vi "FindTreeKey.vi"(8 "error in (no error)":errorcluster, 10 "Key":T3, 11 "Map":T4) -> (0 "error out":errorcluster, 1 "How rotated?":i8[](array[numeric]), 2 "DecisionRecord":T1, 3 "IsFound?":bool)   [LabVIEW 2020]
uses:
  controls/DecisionTree.ctl
  controls/Gameboard Data.ctl
  controls/DecisionTreeRecord.ctl
  controls/Player.ctl
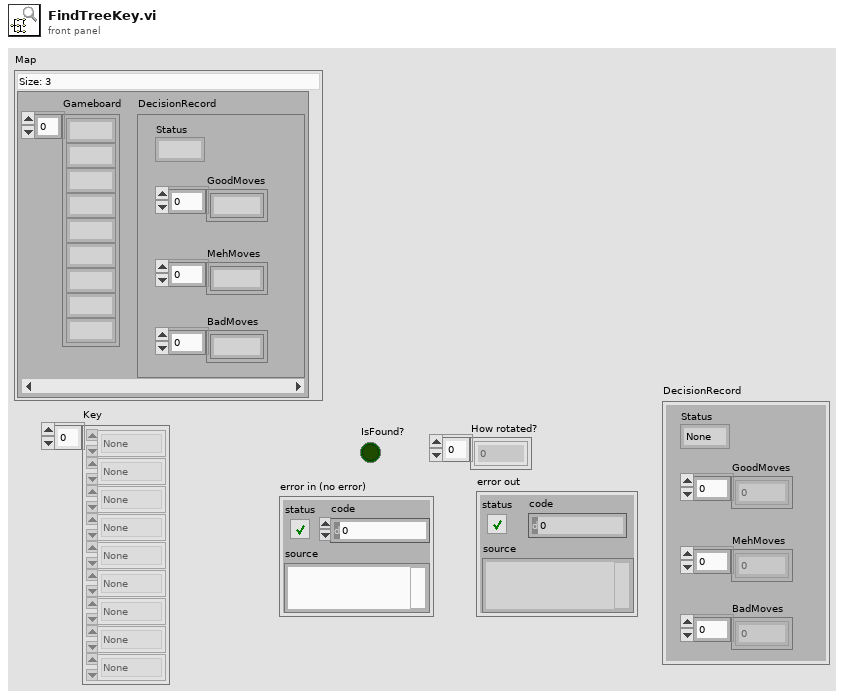
[diagram p1: front panel]
types:
  T1 = typedef "DecisionTreeRecord.ctl" = cluster{"Status":T2, "GoodMoves":i8[], "MehMoves":i8[], "BadMoves":i8[]}
  T2 = typedef "Player.ctl" = enum16{"None", "Player 1", "Player 2"}
  T3 = typedef "Gameboard Data.ctl" = enum16{"None", "Player 1", "Player 2"}[]
  T4 = typedef "DecisionTree.ctl" = map{T3, T1}
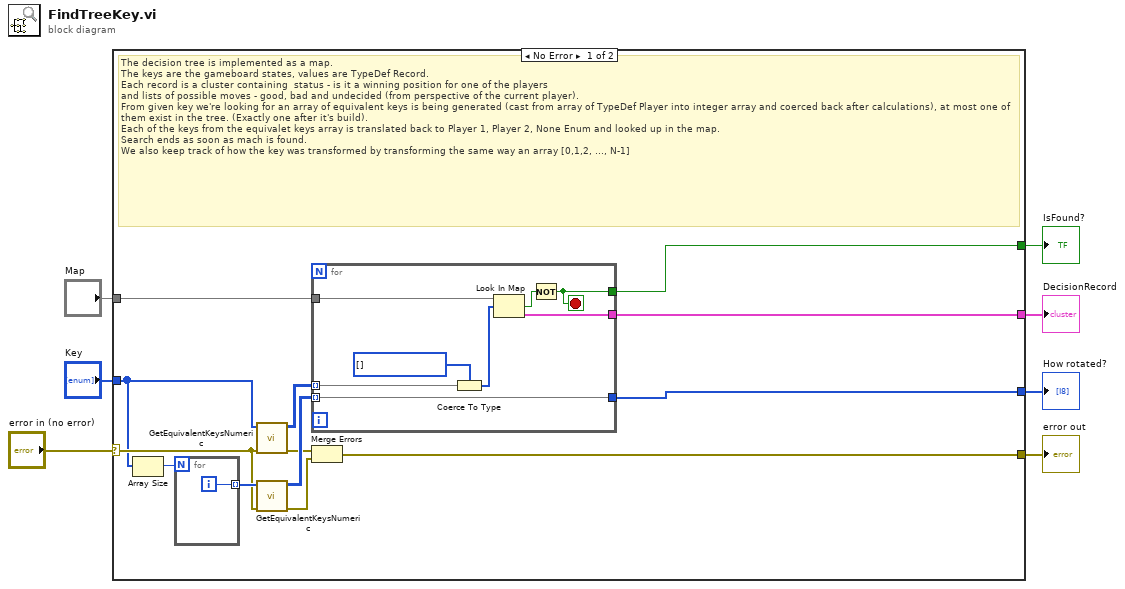
[diagram p0: block diagram]
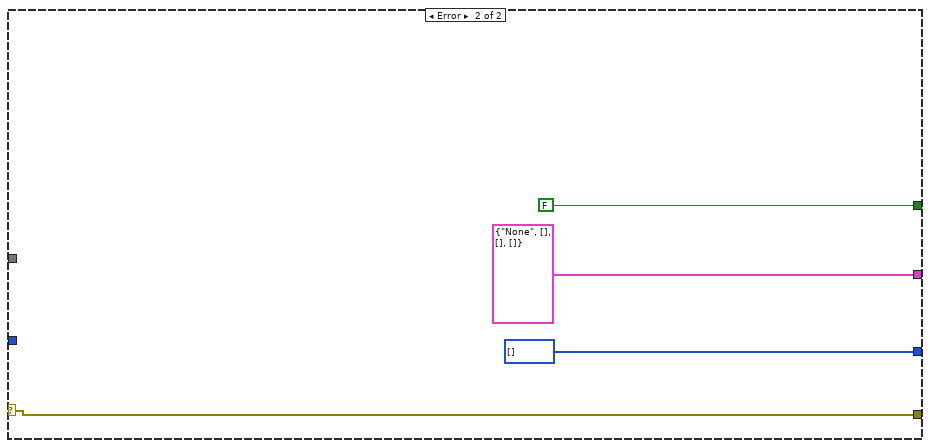
[diagram p2: hidden frame]
diagram:
  n1 = case shown="No Error" "error in (no error)" {
    selector: "error in (no error)" -> [w14 w33]
    tunnel: [w8 w33] -> w6
    tunnel: "Map" -> [w12 _]
    tunnel: "Key" -> [w9 _]
    tunnel: [w20 FALSE] -> w3
    tunnel: [w10 T1 {"Status"=enum."None", "GoodMoves"=[], "MehMoves"=[], "BadMoves"=[]} ("DecisionRecord")] -> w1
    tunnel: [w15 i8[] [] ("KeysEquivalenceClassNumeric")] -> w2
    frame No Error {
      # "The decision tree is implemented as a map. \nThe keys are the gameboard states, values are TypeDef Record.\nEach record is a cluster containing  status - is it a winning position for one of the players \nand lists of possible moves - good, bad and undecided (from perspective of the current player).\nFrom given key we're looking for an array of equivalent keys is being generated (cast from array of TypeDef Player into integer array and coerced back after calculations), at most one of them exist in the tree. (Exactly one after it's build).\nEach of the keys from the equivalet keys array is translated back to Player 1, Player 2, None Enum and looked up in the map. \nSearch ends as soon as mach is found.\nWe also keep track of how the key was transformed by transforming the same way an array [0,1,2, ..., N-1]"
      n2 = Array Size(array=w9) -> (size(s)=w18:i32)
      n3 = for {
        N: w18 -> [_]
        tunnel: [w29] -> w17 mode=indexing
        i -> [w29]
      }
      n4 = call "GetEquivalentKeysNumeric.vi"("error in (no error)"=w14, "KeyNumeric"=w9) -> ("error out"=w13:errorcluster, "KeysEquivalenceClassNumeric"=w11:i8[][])  [unwired: 8 in]
      n5 = call "GetEquivalentKeysNumeric.vi"("error in (no error)"=w14, "KeyNumeric"=w17) -> ("error out"=w19:errorcluster, "KeysEquivalenceClassNumeric"=w16:i8[][])  [unwired: 8 in]
      n6 = for {
        tunnel: [w21] -> w20
        tunnel: w16 -> [w28] mode=indexing
        tunnel: [w28] -> w15
        tunnel: w12 -> [w27]
        tunnel: w11 -> [w22] mode=indexing
        tunnel: [w26] -> w10
        stop <- w21 stop-if-true
        w23 = T2[] [] items=["None", "Player 1", "Player 2"] ("Array")
        n7 = Coerce To Type(0:w22, 1:w23) -> (2:w24:T2[])
        n8 = Look In Map(map=w27, key=w24) -> (key not found?=w25:bool, value=w26:T1)  [unwired: 1 in]
        n9 = Not(x=w25) -> (.not. x?=w21:bool)
      }
      n10 = Merge Errors(w13, w19) -> (w8:errorcluster)
    }
    frame Error {
    }
  }
  "IsFound?" <- w3
  "DecisionRecord" <- w1
  "error out" <- w6
  "How rotated?" <- w2
